vi "RTS Extract Volt Freq.vi"(8 "Error In":errorcluster, 11 "Chamber 1 Socket":string[][](array[string])) -> (0 "Error Out":errorcluster, 3 "Chamber 1":T1={"Voltage 1"=0.0, "Voltage 2"=0.0, "Voltage 3"=0.0, "Voltage 4"=0.0, "Voltage 5"=0.0, "Voltage 6"=0.0, "Voltage 7"=0.0, "Voltage 8"=0.0, "Frequency 1"=0, "Frequency 2"=0, "Frequency 3"=0, "Frequency 4"=0, "Frequency 5"=0, "Frequency 6"=0, "Frequency 7"=0, "Frequency 8"=0, "Ground Leak Relays"={"Ground Leakage 1"=enum."0 - Normal GL", "Ground Leakage 2"=enum."0 - Normal GL", "Ground Leakage 3"=enum."0 - Normal GL", "Ground Leakage 4"=enum."0 - Normal GL", "Ground Leakage 5"=enum."0 - Normal GL", "Ground Leakage 6"=enum."0 - Normal GL", "Ground Leakage 7"=enum."0 - Normal GL", "Ground Leakage 8"=enum."0 - Normal GL"}, "Polarity Selector"={"Station 1"=enum."Ground Neutral", "Station 2"=enum."Ground Neutral", "Station 3"=enum."Ground Neutral", "Station 4"=enum."Ground Neutral", "Station 5"=enum."Ground Neutral", "Station 6"=enum."Ground Neutral", "Station 7"=enum."Ground Neutral", "Station 8"=enum."Ground Neutral"}, "Room Setpoints"={"Room Setpoint Temperature (*RM Dry Set P1)"=90.0, "Room Setpoint Humidity (*RM Hum Set P1)"=20.0, "Room Cool Temperature (*RM Cool Setp 1)"=65.0, "Room Dehum Temperature (*RM De Hum Set P1)"=60.0}} {"Room Setpoints"."Room Dehum Temperature (*RM De Hum Set P1)" min=30.0 max=120.0; "Room Setpoints"."Room Cool Temperature (*RM Cool Setp 1)" min=30.0 max=120.0; "Room Setpoints"."Room Setpoint Humidity (*RM Hum Set P1)" min=5.0 max=98.0; "Room Setpoints"."Room Setpoint Temperature (*RM Dry Set P1)" min=40.0 max=120.0; "Frequency 8" items=["60 Hz", "50 Hz"]; "Frequency 7" items=["60 Hz", "50 Hz"]; "Frequency 6" items=["60 Hz", "50 Hz"]; "Frequency 5" items=["60 Hz", "50 Hz"]; "Frequency 4" items=["60 Hz", "50 Hz"]; "Frequency 3" items=["60 Hz", "50 Hz"]; "Frequency 2" items=["60 Hz", "50 Hz"]; "Frequency 1" items=["60 Hz", "50 Hz"]})   [LabVIEW 2020]
uses:
  Type Definitions/RTS Voltage Frequency Settings.ctl
  Type Definitions/RTS Frequency Selector.ctl
  Drivers/WAGO 750-881/Type Definitions/Wago Ground Leakage Relays.ctl
  Drivers/WAGO 750-881/Type Definitions/Wago Ground Leakage.ctl
  Drivers/WAGO 750-881/Type Definitions/Wago Polarity Selector Relays.ctl
  Drivers/WAGO 750-881/Type Definitions/Wago Polarity Selector.ctl
  Type Definitions/RTS Chamber Temperature Humidity Control.ctl
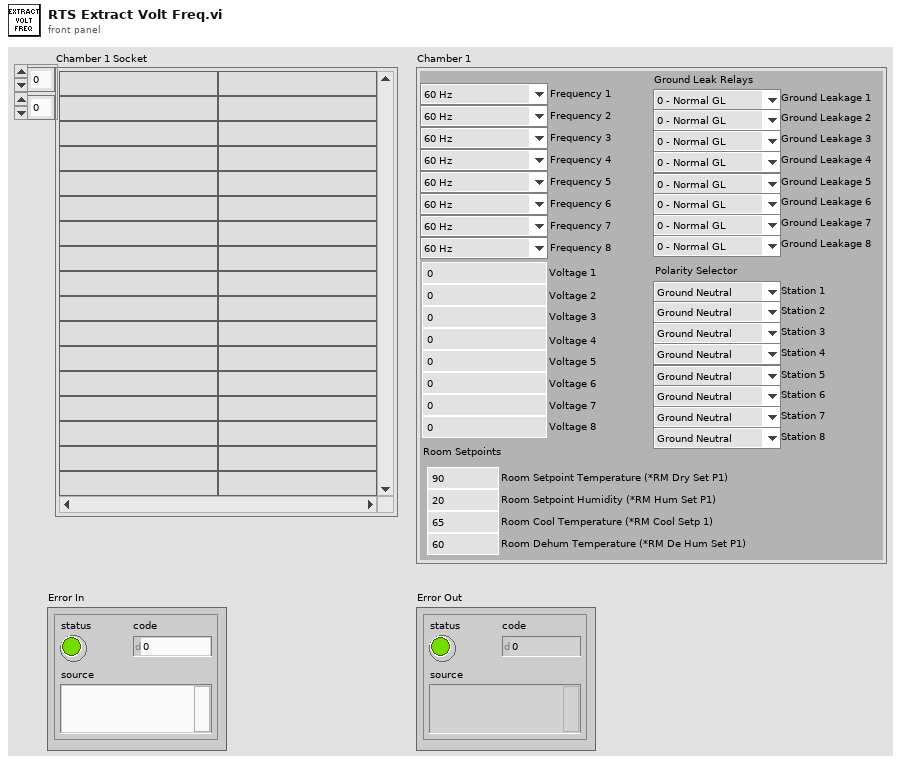
[diagram p1: front panel]
types:
  T1 = typedef "RTS Voltage Frequency Settings.ctl" = cluster{"Voltage 1":dbl, "Voltage 2":dbl, "Voltage 3":dbl, "Voltage 4":dbl, "Voltage 5":dbl, "Voltage 6":dbl, "Voltage 7":dbl, "Voltage 8":dbl, "Frequency 1":T2, "Frequency 2":T2, "Frequency 3":T2, "Frequency 4":T2, "Frequency 5":T2, "Frequency 6":T2, "Frequency 7":T2, "Frequency 8":T2, "Ground Leak Relays":T3, "Polarity Selector":T5, "Room Setpoints":T7}
  T2 = typedef "RTS Frequency Selector.ctl" = u16
  T3 = typedef "Wago Ground Leakage Relays.ctl" = cluster{"Ground Leakage 1":T4, "Ground Leakage 2":T4, "Ground Leakage 3":T4, "Ground Leakage 4":T4, "Ground Leakage 5":T4, "Ground Leakage 6":T4, "Ground Leakage 7":T4, "Ground Leakage 8":T4}
  T4 = typedef "Wago Ground Leakage.ctl" = enum16{"0 - Normal GL", "1 - Measure GL"}
  T5 = typedef "Wago Polarity Selector Relays.ctl" = cluster{"Station 1":T6, "Station 2":T6, "Station 3":T6, "Station 4":T6, "Station 5":T6, "Station 6":T6, "Station 7":T6, "Station 8":T6}
  T6 = typedef "Wago Polarity Selector.ctl" = enum16{"Ground Neutral", "Ground Line"}
  T7 = typedef "RTS Chamber Temperature Humidity Control.ctl" = cluster{"Room Setpoint Temperature (*RM Dry Set P1)":dbl, "Room Setpoint Humidity (*RM Hum Set P1)":dbl, "Room Cool Temperature (*RM Cool Setp 1)":dbl, "Room Dehum Temperature (*RM De Hum Set P1)":dbl}
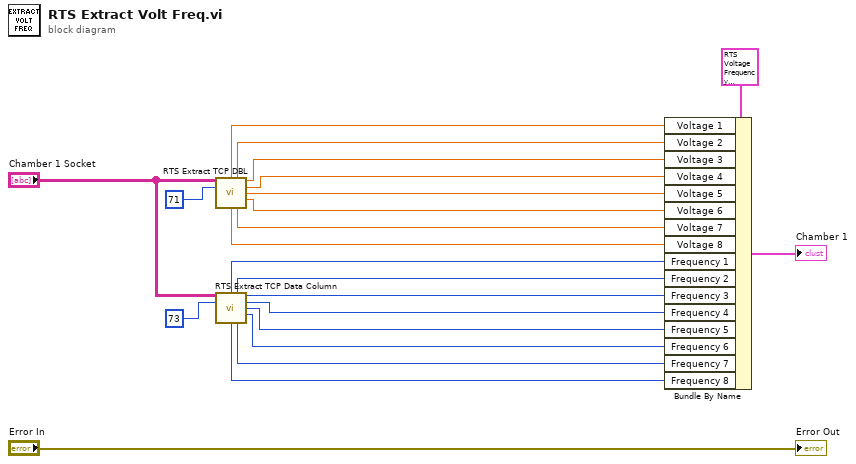
[diagram p0: block diagram]
diagram:
  n1 = call "RTS Extract TCP DBL.vi"("Chamber 1 Socket"="Chamber 1 Socket", "Extract Column"=71) -> ("Station 1"=w9:dbl, "Station 2"=w8:dbl, "Station 3"=w7:dbl, "Station 4"=w6:dbl, "Station 5"=w5:dbl, "Station 6"=w4:dbl, "Station 8"=w2:dbl, "Station 7"=w3:dbl)  [unwired: 5 in, 1 out]
  n2 = call "RTS Extract TCP Data Column.vi"("Chamber 1 Socket"="Chamber 1 Socket", "Extract Column"=73) -> ("Station 1"=w17:i32, "Station 2"=w16:i32, "Station 3"=w15:i32, "Station 4"=w14:i32, "Station 5"=w13:i32, "Station 6"=w12:i32, "Station 8"=w10:i32, "Station 7"=w11:i32)  [unwired: 5 in, 1 out]
  n3 = Bundle By Name(cluster=T1 {"Voltage 1"=0.0, "Voltage 2"=0.0, "Voltage 3"=0.0, "Voltage 4"=0.0, "Voltage 5"=0.0, "Voltage 6"=0.0, "Voltage 7"=0.0, "Voltage 8"=0.0, "Frequency 1"=0, "Frequency 2"=0, "Frequency 3"=0, "Frequency 4"=0, "Frequency 5"=0, "Frequency 6"=0, "Frequency 7"=0, "Frequency 8"=0, "Ground Leak Relays"={"Ground Leakage 1"=enum."0 - Normal GL", "Ground Leakage 2"=enum."0 - Normal GL", "Ground Leakage 3"=enum."0 - Normal GL", "Ground Leakage 4"=enum."0 - Normal GL", "Ground Leakage 5"=enum."0 - Normal GL", "Ground Leakage 6"=enum."0 - Normal GL", "Ground Leakage 7"=enum."0 - Normal GL", "Ground Leakage 8"=enum."0 - Normal GL"}, "Polarity Selector"={"Station 1"=enum."Ground Neutral", "Station 2"=enum."Ground Neutral", "Station 3"=enum."Ground Neutral", "Station 4"=enum."Ground Neutral", "Station 5"=enum."Ground Neutral", "Station 6"=enum."Ground Neutral", "Station 7"=enum."Ground Neutral", "Station 8"=enum."Ground Neutral"}, "Room Setpoints"={"Room Setpoint Temperature (*RM Dry Set P1)"=90.0, "Room Setpoint Humidity (*RM Hum Set P1)"=20.0, "Room Cool Temperature (*RM Cool Setp 1)"=65.0, "Room Dehum Temperature (*RM De Hum Set P1)"=60.0}} ("Chamber 2"), "Voltage 1"=w9, "Voltage 2"=w8, "Voltage 3"=w7, "Voltage 4"=w6, "Voltage 5"=w5, "Voltage 6"=w4, "Voltage 7"=w3, "Voltage 8"=w2, "Frequency 1"=w17, "Frequency 2"=w16, "Frequency 3"=w15, "Frequency 4"=w14, "Frequency 5"=w13, "Frequency 6"=w12, "Frequency 7"=w11, "Frequency 8"=w10) -> (→"Chamber 1":T1)
  "Error Out" <- "Error In"
